vi "writeU16FIFO.vi"(8 "error in (no error)":errorcluster, 9 "Timeout":i32, 10 "Data":u16[](array[numeric]), 11 "ModbusSubnetCTxDataFIFO in":refnum<class "ModbusSubnetCTxDataFIFO.lvclass">) -> (0 "error out":errorcluster, 2 "ElementsRemaining":u32, 3 "ModbusSubnetCTxDataFIFO out":refnum<class "ModbusSubnetCTxDataFIFO.lvclass">)   [LabVIEW 2016, in "ModbusSubnetCTxDataFIFO.lvclass"]
uses:
  ModbusSubnetCTxDataFIFO.lvclass
  FPGA/FPGA.lvclass
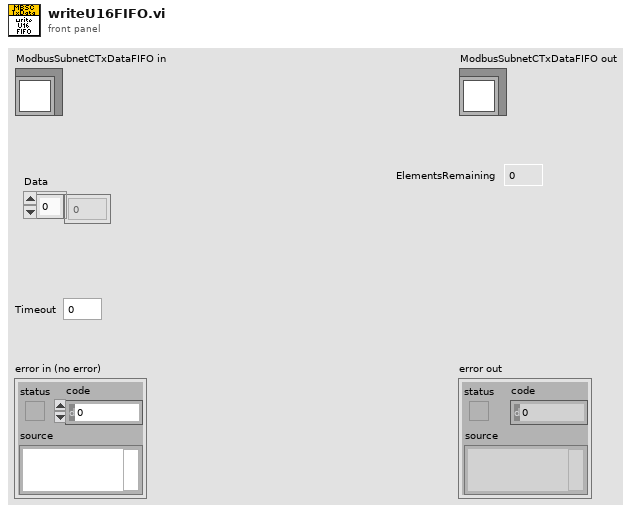
[diagram p1: front panel]
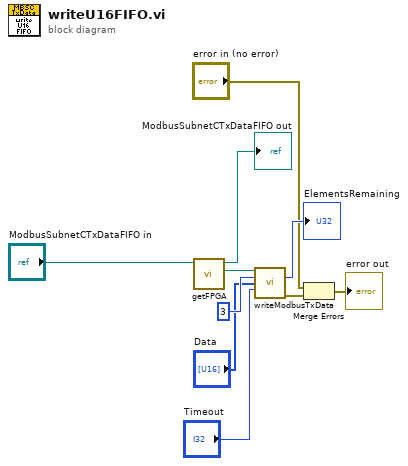
[diagram p0: block diagram]
diagram:
  n1 = call "getFPGA.vi"("ModbusSubnetCTxDataFIFO in"="ModbusSubnetCTxDataFIFO in") -> ("FPGA"=w9:refnum<class "FPGA.lvclass">, "ModbusSubnetCTxDataFIFO out"=→"ModbusSubnetCTxDataFIFO out":refnum<class "ModbusSubnetCTxDataFIFO.lvclass">)  [unwired: 9 in]
  n2 = call "writeModbusTxData.vi"("FPGA in"=w9, 5:u16 3 ("Subnet"), 7:"Data", "Timeout (ms)"="Timeout") -> ("Empty Elements Remaining"=→"ElementsRemaining":u32, "error out"=w2:errorcluster)  [unwired: 9 in, 1 out]
  n3 = Merge Errors("error in (no error)", w2) -> (→"error out":errorcluster)
